vi "EasterEgg.vi"() -> ()   [LabVIEW 2014]
uses:
  <vilib>/Platform/TimedLoop/XDataNode/timing_clust.ctl
  <vilib>/Platform/TimedLoop/XDataNode/nitl_modes.ctl
  <vilib>/Platform/TimedLoop/XDataNode/wakeup.ctl
  <vilib>/Platform/TimedLoop/XDataNode/XDataNode.xnode
  <vilib>/Platform/TimedLoop/XDataNode/XDNodeRunTimeDep.lvlib
panel:
  out "error out":errorcluster
  in  "Close":bool
  out "2D Picture":picture
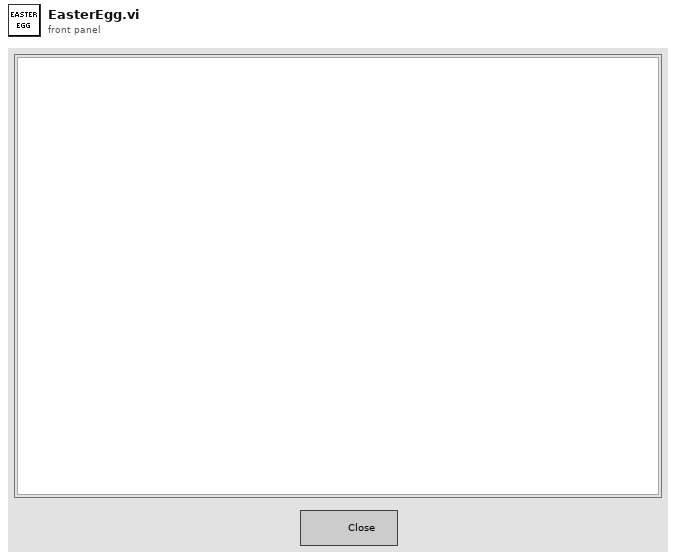
[diagram p1: front panel]
types:
  T1 = typedef "XDNodeRunTimeDep.lvlib/timing_clust.ctl" = cluster{"Expected End [f-1]":u64, "Actual End [f-1]":u64, "Finished Late? [f-1]":bool, "Expected End [i-1]":u64, "Actual End [i-1]":u64, "Finished Late? [i-1]":bool, "Expected Start [i]":u64, "Actual Start [i]":u64, "Expected Start [f]":u64, "Actual Start [f]":u64, "Source Name":string, "Structure Name":string, "Period":i64, "Deadline":i64, "Offset":i64, "Start":i64, "Priority":i32, "Timeout":i32, "Mode":T2, "Wakeup Reason":T3, "Error":errorcluster, "Source Type":string, "Secondary Source Type":string, "Global End Time":u64, "Global Start Time":u64, "Frame Duration":u64, "Iteration Duration":u64, "Assigned CPU":i32, "I/O Scan Engine Mode":u32}
  T2 = typedef "XDNodeRunTimeDep.lvlib/nitl_modes.ctl" = enum32{"No Change", "Process missed periods, maintain original phase", "Discard missed periods, maintain original phase", "Process missed periods, ignore original phase", "Discard missed periods, ignore original phase"}
  T3 = typedef "XDNodeRunTimeDep.lvlib/wakeup.ctl" = enum32{"Normal", "Aborted", "Asynchronous wakeup", "Timing source error", "Timed loop error", "Timeout"}
  T4 = typedef "imagedata.ctl" = cluster{"image type":i32, "image depth":i32, "image":u8[], "mask":u8[], "colors":u32[], "Rectangle":cluster{"left":i16, "top":i16, "right":i16, "bottom":i16}}
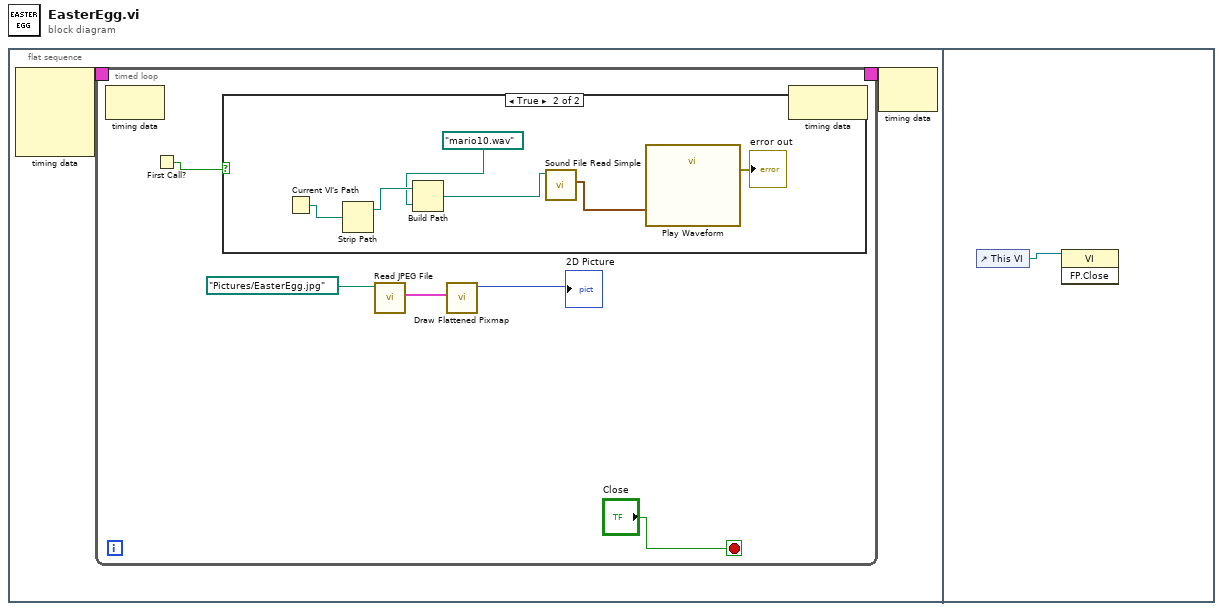
[diagram p0: block diagram]
diagram:
  n1 = flat-sequence {
    frame #0 {
      n2 = node-c288() -> (w2:T1)  [unwired: 4 in]
      n3 = timed-loop {
        timing: w2 -> [_]
        timing-out: [_] -> w1
        stop <- "Close" stop-if-true
        n4 = node-c288() -> ()  [unwired: 1 in, 1 out]
        n5 = First Call?() -> (First Call?: T/F=w3:bool)
        n6 = case shown="True" w3 {
          frame False {
          }
          frame True {
            n7 = Current VI's Path() -> (path=w14:path)
            n8 = Strip Path(path=w14) -> (stripped path=w13:path)  [unwired: 1 out]
            n9 = Build Path(base path=w13, name or relative path=path "mario10.wav") -> (appended path=w11:path)
            n10 = call <vilib>:"Sound File Read Simple.vi"("path"=w11) -> ("data"=w15:waveform(dbl)[])  [unwired: 7 in, 3 out]
            n11 = call "Play Waveform"("Data"=w15) -> ("error out"=→"error out":errorcluster)  [unwired: 18 in]
          }
        }
        n12 = call <vilib>:"Read JPEG File.vi"("path to JPEG file"=path "Pictures/EasterEgg.jpg") -> ("image data"=w6:T4)  [unwired: 8 in, 2 out]
        n13 = call <vilib>:"Draw Flattened Pixmap.vi"("image data"=w6) -> ("new picture"=→"2D Picture":picture)  [unwired: 8 in]
        n14 = node-c288() -> ()  [unwired: 1 in, 1 out]
      }
      n15 = node-c288(w1) -> ()  [unwired: 1 out]
    }
    frame #1 {
      n16 = control-ref of="This VI"() -> (w18:refnum<vi>)
      n17 = invoke class="VI" method="FP.Close"(reference=w18) -> ()  [unwired: 2 in, 3 out]
    }
  }
